vi "Spartan HTTP Send Log Message.vi"(7 "message":string) -> ()   [LabVIEW 2011]
uses:
  Spartan HTTP Server Globals.vi
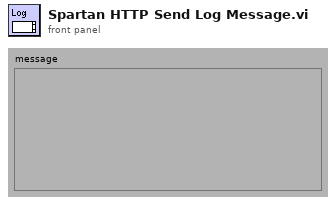
[diagram p1: front panel]
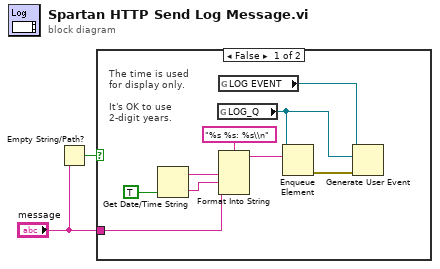
[diagram p0: block diagram]
diagram:
  n1 = Empty String/Path?(string/path="message") -> (empty?=w1:bool)
  n2 = case shown="False" w1 {
    tunnel: "message" -> [w11 _]
    frame False {
      # "The time is used for display only.\n\nIt's OK to use 2-digit years."
      n3 = Get Date/Time String(want seconds? (F)=TRUE) -> (date string=w8:string, time string=w9:string)  [unwired: 2 out]
      n4 = global read "Spartan HTTP Server Globals.vi" "LOG_Q"() -> (w5:refnum<queue>)
      n5 = global read "Spartan HTTP Server Globals.vi" "LOG EVENT"() -> (w3:refnum<user-event>)
      n6 = Format Into String(format string="%s %s: %s\\n", w8, w9, w11) -> (resulting string=w10:string)  [unwired: 2 in, 1 out]
      n7 = Enqueue Element(queue=w5, element=w10) -> (error out=w4:errorcluster)  [unwired: 1 in, 3 out]
      n8 = Generate User Event(user event=w3, event data cluster=w5, error in=w4) -> ()  [unwired: 2 out]
    }
    frame True {
    }
  }
